vi "LanchAngleAndSpeed.vi"(2 "g":dbl, 3 "entry angle":dbl, 4 "height":dbl, 5 "horizontal distance":dbl) -> (0 "speed":dbl, 1 "angle":dbl)   [LabVIEW 2011]
uses:
  <vilib>/express/express arith-compare/Formula/XNode/ExpressFormulaBlockNode.xnode
panel:
  # "b"
  # "angle - degrees\nb - degrees\nh - meters\nd - meters\ng - m/s^2\nspeed - m/s"
  # "V"
  # "h"
  # "angle"
  # "d"
  # "d - horizontal distance\nh - height\nb - entry angle\nV - speed"
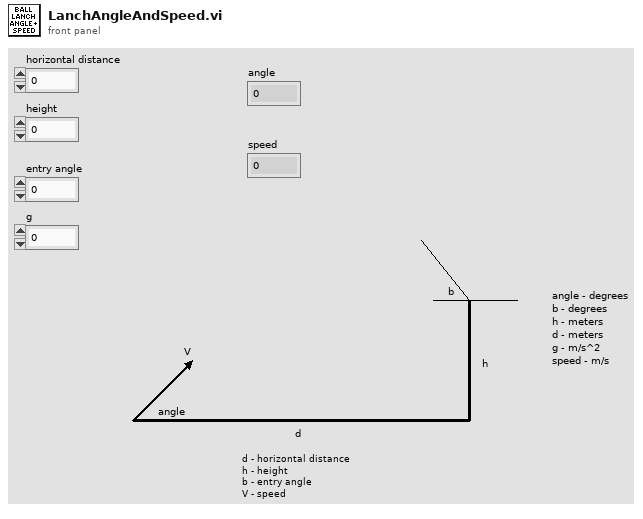
[diagram p1: front panel]
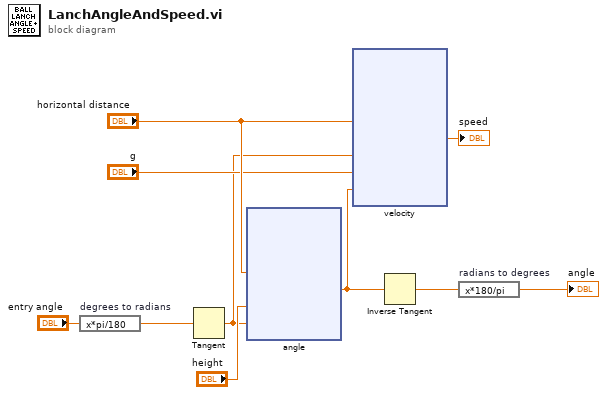
[diagram p0: block diagram]
diagram:
  n1 = expression code="x*pi/180" "degrees to radians"("entry angle") -> (w4:dbl)
  n2 = Tangent(1:w4) -> (0:w3:dbl)
  n3 = xnode "angle"("d"="horizontal distance", "h"="height", "tb"=w3) -> ("Result"=w2:dbl)  [unwired: 1 in, 1 out]
  n4 = xnode "velocity"("d"="horizontal distance", "tb"=w3, "g"="g", "ta"=w2) -> ("Result"=→"speed":dbl)  [unwired: 1 in, 1 out]
  n5 = Inverse Tangent(1:w2) -> (0:w1:dbl)
  n6 = expression code="x*180/pi" "radians to degrees"(w1) -> (→"angle":dbl)
